vi "Create (Dimensions).vi"(8 "error in (no error)":errorcluster, 10 "Dimensions":i32[](array[numeric]), 11 "U16 array in":u16[](array[numeric])) -> (0 "error out":errorcluster, 3 "Uint16Array out":refnum<class "Uint16Array.lvclass">)   [LabVIEW 2013, in "MDSplus.lvlib" / "Uint16Array.lvclass"]
uses:
  <vilib>/MDSplus/Classes/Data_Class/Array_Class/Uint16Array_Class/Uint16Array.lvclass
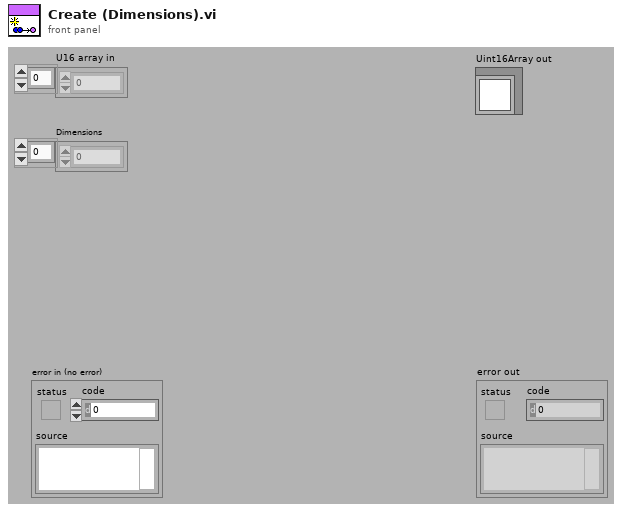
[diagram p1: front panel]
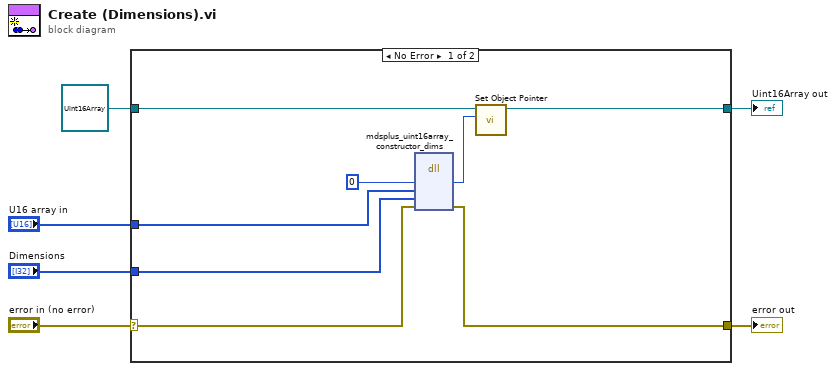
[diagram p0: block diagram]
diagram:
  n1 = case shown="No Error" "error in (no error)" {
    selector: "error in (no error)" -> [w12 w16]
    tunnel: [w7 w16] -> w5
    tunnel: [w10 w15] -> w3
    tunnel: refnum<class "Uint16Array.lvclass"> refnum ("Float32 in") -> [w11 w15]
    tunnel: "U16 array in" -> [w9 _]
    tunnel: "Dimensions" -> [w8 _]
    frame No Error {
      n2 = dll-call lib="MDSobjectsLVShr" fn="mdsplus_uint16array_constructor_dims"("lvUint16ArrayPtrOut"=i64 0 ("lvTreePtr"), "lvUShtArrHdlIn"=w9, "lvIntArrHdlIn"=w8, "error"=w12) -> ("lvUint16ArrayPtrOut"=w13:i64, "error"=w7:errorcluster)  [unwired: 6 in, 2 out]
      n3 = call-dynamic "Set Object Pointer.vi"("Object Pointer"=w13, "Data in"=w11) -> ("Data out"=w10:refnum<class "Uint16Array.lvclass">)  [unwired: 9 in]
    }
    frame Error {
    }
  }
  "error out" <- w5
  "Uint16Array out" <- w3
